vi "fft of the signal.vi"() -> ()   [LabVIEW 2017]
uses:
  <vilib>/Analysis/2dsp.llb/Real FFT.vi
  <vilib>/Analysis/NI_AALPro.lvlib
panel:
  out "main signal":waveform(dbl)[](graph) caption="Filtered Signal"
  out "fft imaginary":dbl[](graph) caption="Filtered Signal"
  out "fft real":dbl[](graph) caption="Filtered Signal"
  out "y":dbl[](array[numeric])
  out "x":dbl[](array[numeric])
  in  "path 3":path
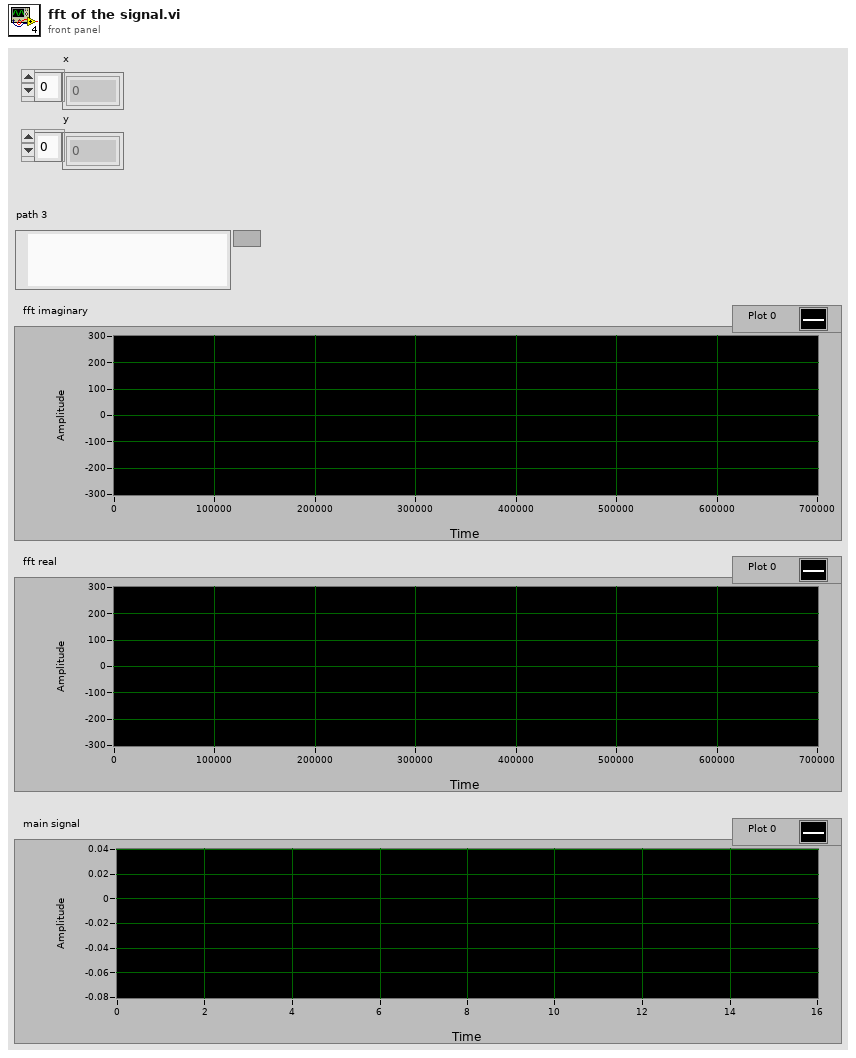
[diagram p1: front panel]
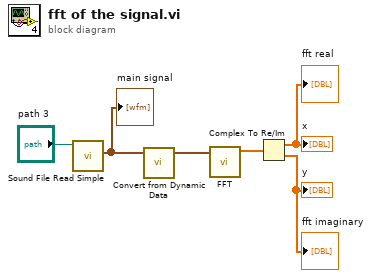
[diagram p0: block diagram]
diagram:
  n1 = call <vilib>:"Sound File Read Simple.vi"("path"="path 3") -> ("data"=w2:waveform(dbl)[])  [unwired: 7 in, 3 out]
  "main signal" <- w2
  n2 = call "Convert from Dynamic Data"("Dynamic Data Type"=w2) -> ("Waveform"=w1:waveform(dbl))  [unwired: 3 in]
  n3 = call-poly <vilib>:"FFT.vi"("X"=w1) -> ("FFT {X}"=w3:cdb[])  [unwired: 9 in, 1 out]
  n4 = Complex To Re/Im(x + iy=w3) -> (x=→"x" →"fft real":dbl[], y=→"y" →"fft imaginary":dbl[])
